vi "FTW-JSON-Object-GetElement-SerializedObject.vi"(0 "JSON":refnum<class "FTW-Container.lvclass">, 5 "Key":string, 7 "Default Value":string, 9 "Consume Value":bool, 11 "error in":errorcluster) -> (4 "JSON out":refnum<class "FTW-Container.lvclass">, 6 "JSON Element Type":T1, 8 "Value":string, 10 "Found":bool, 15 "error out":errorcluster)   [LabVIEW 2015]
uses:
  container/FTW-Container.lvclass
  FTW-JSON-Type.ctl
panel:
  # "Inputs"
  # "Outputs"
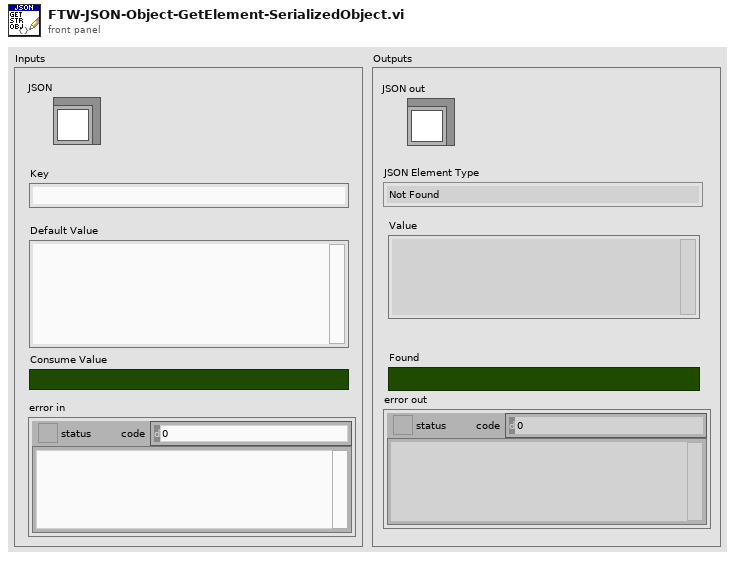
[diagram p1: front panel]
types:
  T1 = typedef "FTW-JSON-Type.ctl" = enum8{"Not Found", "Object", "Array", "String", "Number", "Boolean", "null"}
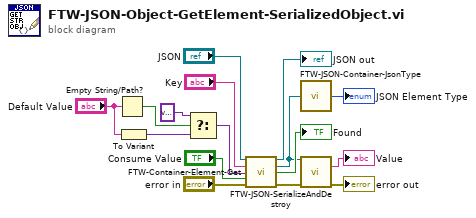
[diagram p0: block diagram]
diagram:
  n1 = Empty String/Path?(string/path="Default Value") -> (empty?=w4:bool)
  n2 = To Variant(anything="Default Value") -> (Variant=w3:variant)
  n3 = Select(t=variant, s=w4, f=w3) -> (s? t:f=w1:variant)
  n4 = call "FTW-Container-Element-Get.vi"("FTW-Container In"="JSON", "Element Name"="Key", "Default Value"=w1, "Delete?"="Consume Value", "error in"="error in") -> ("FTW-Container Out"=→"JSON out":refnum<class "FTW-Container.lvclass">, "Element Out"=w7:refnum<class "FTW-Container.lvclass">, "Found"=→"Found":bool, "error out"=w11:errorcluster)  [unwired: 7 in]
  n5 = call "FTW-JSON-Container-JsonType.vi"("Container"=w7) -> ("JSON Element Type"=→"JSON Element Type":T1)  [unwired: 14 in]
  n6 = call "FTW-JSON-SerializeAndDestroy.vi"("JSON"=w7, "error in"=w11) -> ("JSON String (UTF-8)"=→"Value":string, "error out"=→"error out":errorcluster)  [unwired: 12 in]
